vi "search signals worksheet MPB.vi"() -> ()   [LabVIEW 2020]
panel:
  out "path not found":bool
  in  "signal/tag name":string="RX_deltatime"
  out "full path name":string
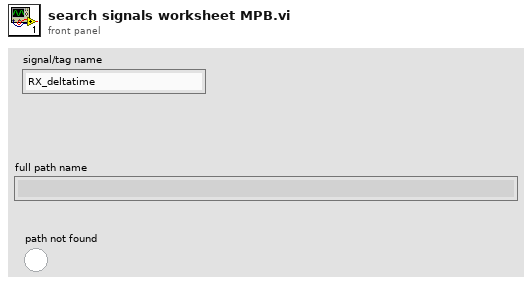
[diagram p1: front panel]
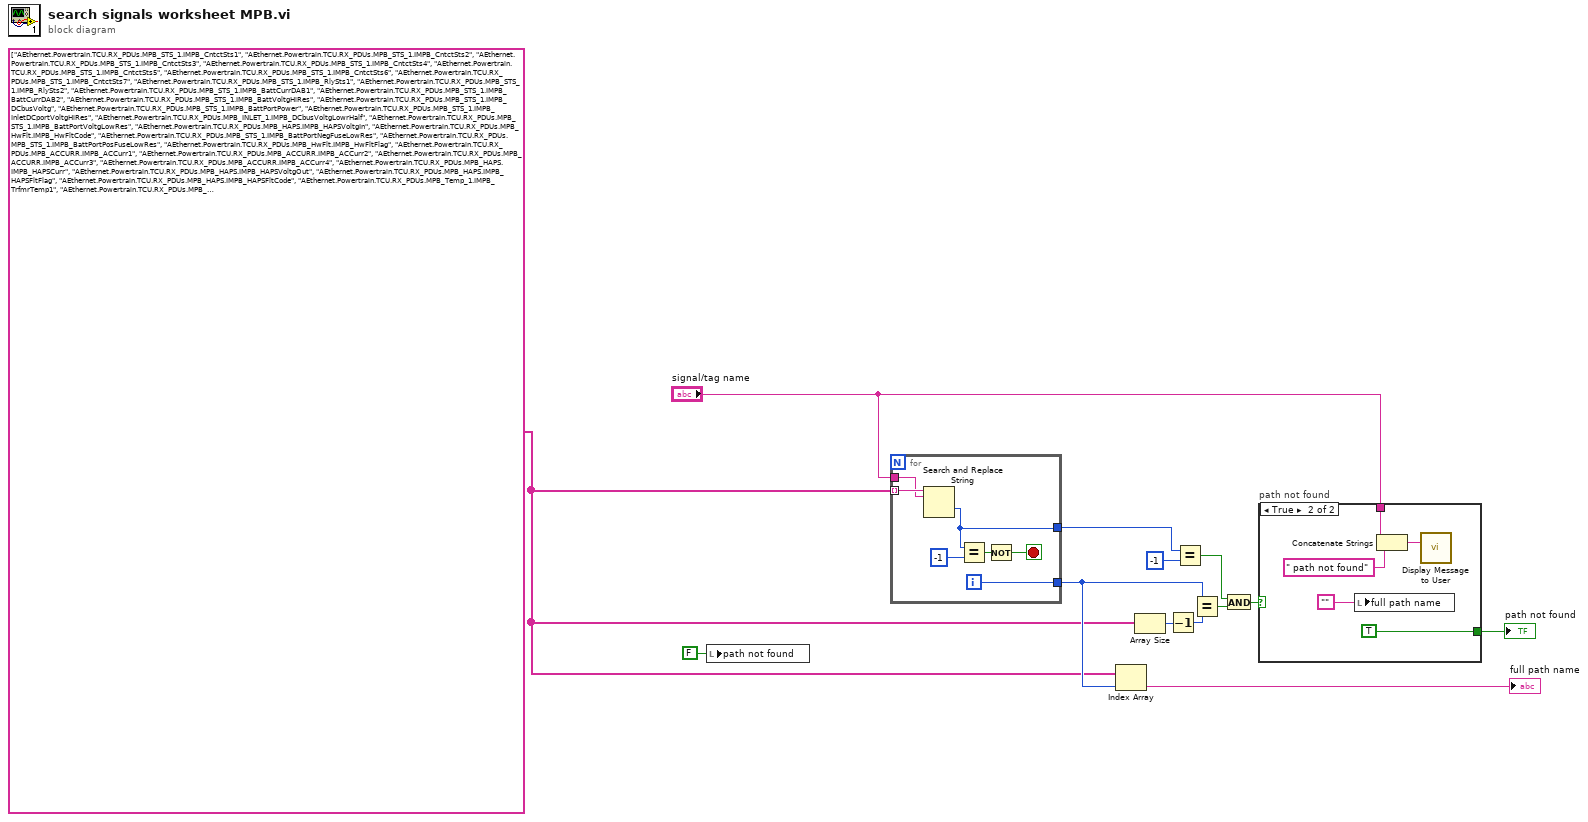
[diagram p0: block diagram]
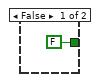
[diagram p2: hidden frame]
diagram:
  w1 = string[] ["AEthernet.Powertrain.TCU.RX_PDUs.MPB_STS_1.IMPB_CntctSts1", "AEthernet.Powertrain.TCU.RX_PDUs.MPB_STS_1.IMPB_CntctSts2", "AEthernet.Powertrain.TCU.RX_PDUs.MPB_STS_1.IMPB_CntctSts3", "AEthernet.Powertrain.TCU.RX_PDUs.MPB_STS_1.IMPB_CntctSts4", "AEthernet.Powertrain.TCU.RX_PDUs.MPB_STS_1.IMPB_CntctSts5", "AEthernet.Powertrain.TCU.RX_PDUs.MPB_STS_1.IMPB_CntctSts6", "AEthernet.Powertrain.TCU.RX_PDUs.MPB_STS_1.IMPB_CntctSts7", "AEthernet.Powertrain.TCU.RX_PDUs.MPB_STS_1.IMPB_RlySts1", "AEthernet.Powertrain.TCU.RX_PDUs.MPB_STS_1.IMPB_RlySts2", "AEthernet.Powertrain.TCU.RX_PDUs.MPB_STS_1.IMPB_BattCurrDAB1", "AEthernet.Powertrain.TCU.RX_PDUs.MPB_STS_1.IMPB_BattCurrDAB2", "AEthernet.Powertrain.TCU.RX_PDUs.MPB_STS_1.IMPB_BattVoltgHiRes", "AEthernet.Powertrain.TCU.RX_PDUs.MPB_STS_1.IMPB_DCbusVoltg", "AEthernet.Powertrain.TCU.RX_PDUs.MPB_STS_1.IMPB_BattPortPower", "AEthernet.Powertrain.TCU.RX_PDUs.MPB_STS_1.IMPB_InletDCportVoltgHiRes", "AEthernet.Powertrain.TCU.RX_PDUs.MPB_INLET_1.IMPB_DCbusVoltgLowrHalf", "AEthernet.Powertrain.TCU.RX_PDUs.MPB_STS_1.IMPB_BattPortVoltgLowRes", "AEthernet.Powertrain.TCU.RX_PDUs.MPB_HAPS.IMPB_HAPSVoltgIn", "AEthernet.Powertrain.TCU.RX_PDUs.MPB_HwFlt.IMPB_HwFltCode", "AEthernet.Powertrain.TCU.RX_PDUs.MPB_STS_1.IMPB_BattPortNegFuseLowRes", "AEthernet.Powertrain.TCU.RX_PDUs.MPB_STS_1.IMPB_BattPortPosFuseLowRes", "AEthernet.Powertrain.TCU.RX_PDUs.MPB_HwFlt.IMPB_HwFltFlag", "AEthernet.Powertrain.TCU.RX_PDUs.MPB_ACCURR.IMPB_ACCurr1", "AEthernet.Powertrain.TCU.RX_PDUs.MPB_ACCURR.IMPB_ACCurr2", "AEthernet.Powertrain.TCU.RX_PDUs.MPB_ACCURR.IMPB_ACCurr3", "AEthernet.Powertrain.TCU.RX_PDUs.MPB_ACCURR.IMPB_ACCurr4", "AEthernet.Powertrain.TCU.RX_PDUs.MPB_HAPS.IMPB_HAPSCurr", "AEthernet.Powertrain.TCU.RX_PDUs.MPB_HAPS.IMPB_HAPSVoltgOut", "AEthernet.Powertrain.TCU.RX_PDUs.MPB_HAPS.IMPB_HAPSFltFlag", "AEthernet.Powertrain.TCU.RX_PDUs.MPB_HAPS.IMPB_HAPSFltCode", "AEthernet.Powertrain.TCU.RX_PDUs.MPB_Temp_1.IMPB_TrfmrTemp1", "AEthernet.Powertrain.TCU.RX_PDUs.MPB_Temp_1.IMPB_TrfmrTemp2", "AEthernet.Powertrain.TCU.RX_PDUs.MPB_STS_1.IMPB_InletACportVoltgHiRes", "AEthernet.Powertrain.TCU.RX_PDUs.MPB_INLET_1.IMPB_DCbusVoltgUpprHalf", "AEthernet.Powertrain.TCU.RX_PDUs.MPB_STS_1.IMPB_HeatgActv", "AEthernet.Powertrain.TCU.RX_PDUs.MPB_INLET_2.IMPB_InletACportEgy", "AEthernet.Powertrain.TCU.RX_PDUs.MPB_STS_1.IMPB_InletACportFuseLowRes", "AEthernet.Powertrain.TCU.RX_PDUs.MPB_STS_1.IMPB_InletDCportPosLowRes", "AEthernet.Powertrain.TCU.RX_PDUs.MPB_STS_1.IMPB_InletDCportNegLowRes"]
  n1 = local write "path not found"(FALSE ("path not found")) -> ()
  n2 = for {
    tunnel: w1 -> [w20] mode=indexing
    tunnel: "signal/tag name" -> [w19]
    tunnel: [w15] -> w12
    tunnel: [w14] -> w8
    i -> [w15]
    stop <- w16 stop-if-true
    n3 = Search and Replace String(input string=w20, search string=w19) -> (offset past replacement=w14:i32)  [unwired: 6 in, 3 out]
    n4 = Equal?(x=w14, y=-1) -> (x = y?=w17:bool)
    n5 = Not(x=w17) -> (.not. x?=w16:bool)
  }
  n6 = Index Array(array=w1, index=w12) -> (element=→"full path name":string)
  n7 = Array Size(array=w1) -> (size(s)=w13:i32)
  n8 = Decrement(x=w13) -> (x-1=w11:i32)
  n9 = Equal?(x=w8, y=-1) -> (x = y?=w6:bool)
  n10 = Equal?(x=w12, y=w11) -> (x = y?=w5:bool)
  n11 = And(x=w6, y=w5) -> (x .and. y?=w4:bool)
  n12 = case "path not found" shown="True" w4 {
    tunnel: "signal/tag name" -> [_ w26]
    tunnel: [FALSE TRUE] -> w3
    frame False {
    }
    frame True {
      n13 = local write "full path name"("") -> ()
      n14 = Concatenate Strings(w26, " path not found" ("string")) -> (w25:string)
      n15 = call "Display Message to User"("Message"=w25) -> ()  [unwired: 9 in, 2 out]
    }
  }
  "path not found" <- w3
